vi "Login.vi"() -> ()   [LabVIEW 2015]
uses:
  <userlib>/QMH/Message Queue/Support/RunType.ctl
  <userlib>/QMH/Message Queue/Support/Enqueue Message (Single).vi
  <userlib>/QMH/Message Queue/Support/Enqueue Message (Array).vi
  <vilib>/Utility/error.llb/Error Cluster From Error Code.vi
  <userlib>/QMH/Message Queue/Support/Run Module(ref).vi
  <vilib>/ErrorRing/Error Ring.xnode
  <userlib>/QMH/User Event - Stop/User Event - Stop.lvlib
  <userlib>/QMH/Message Queue/Message Queue.lvlib
panel:
  in  "Authority":u16(ring) items=["学生", "老师"]
  in  "Login":bool
  in  "PassWord":string
  in  "用户名":string
  in  "Exit":bool
  in  "HostThread":variant
  # "权限 :"
  # "用户名 :"
  # "密码 :"
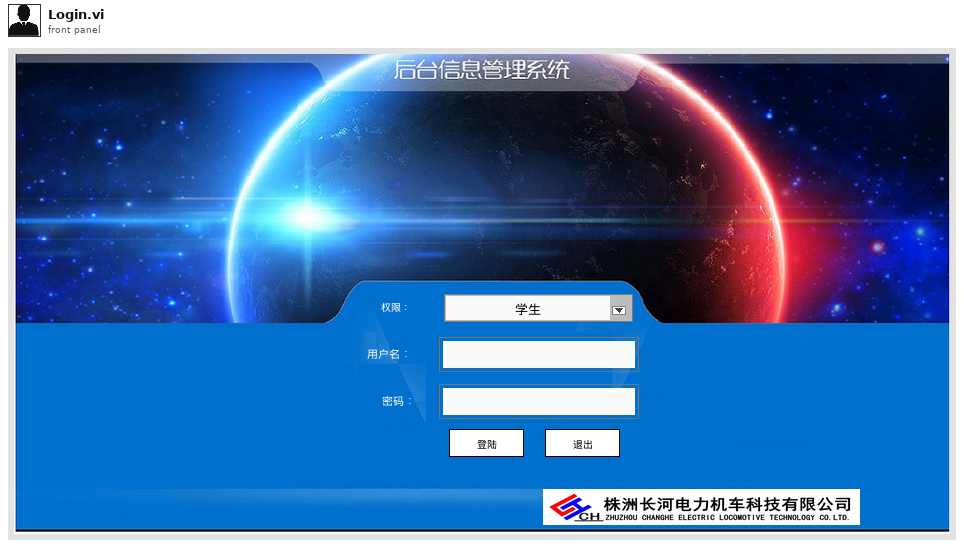
[diagram p1: front panel]
types:
  T1 = cluster{"Controls":cluster{"Exit":refnum<vi>, "Authority":refnum<vi>, "用户名":refnum<vi>, "密码":refnum<vi>}, "Thread":cluster{"ThisQ":string, "ThisVI":refnum<vi>, "HostQ":string, "HostRef":refnum<vi>, "SlavesQ":string[], "SlavesRef":refnum<vi>[]}, "Data":cluster{"Replace":bool}, "User":cluster{"Name":string}, "result?":bool, "Authority":u16}
  T2 = typedef "Message Queue.lvlib/RunType.ctl" = enum16{"Embeded", "Standard", "Hidden", "Minimized", "Maximzed", "RealTime"}
  T3 = cluster{"用户名":refnum<vi>, "密码":refnum<vi>, "Authority":refnum<vi>}
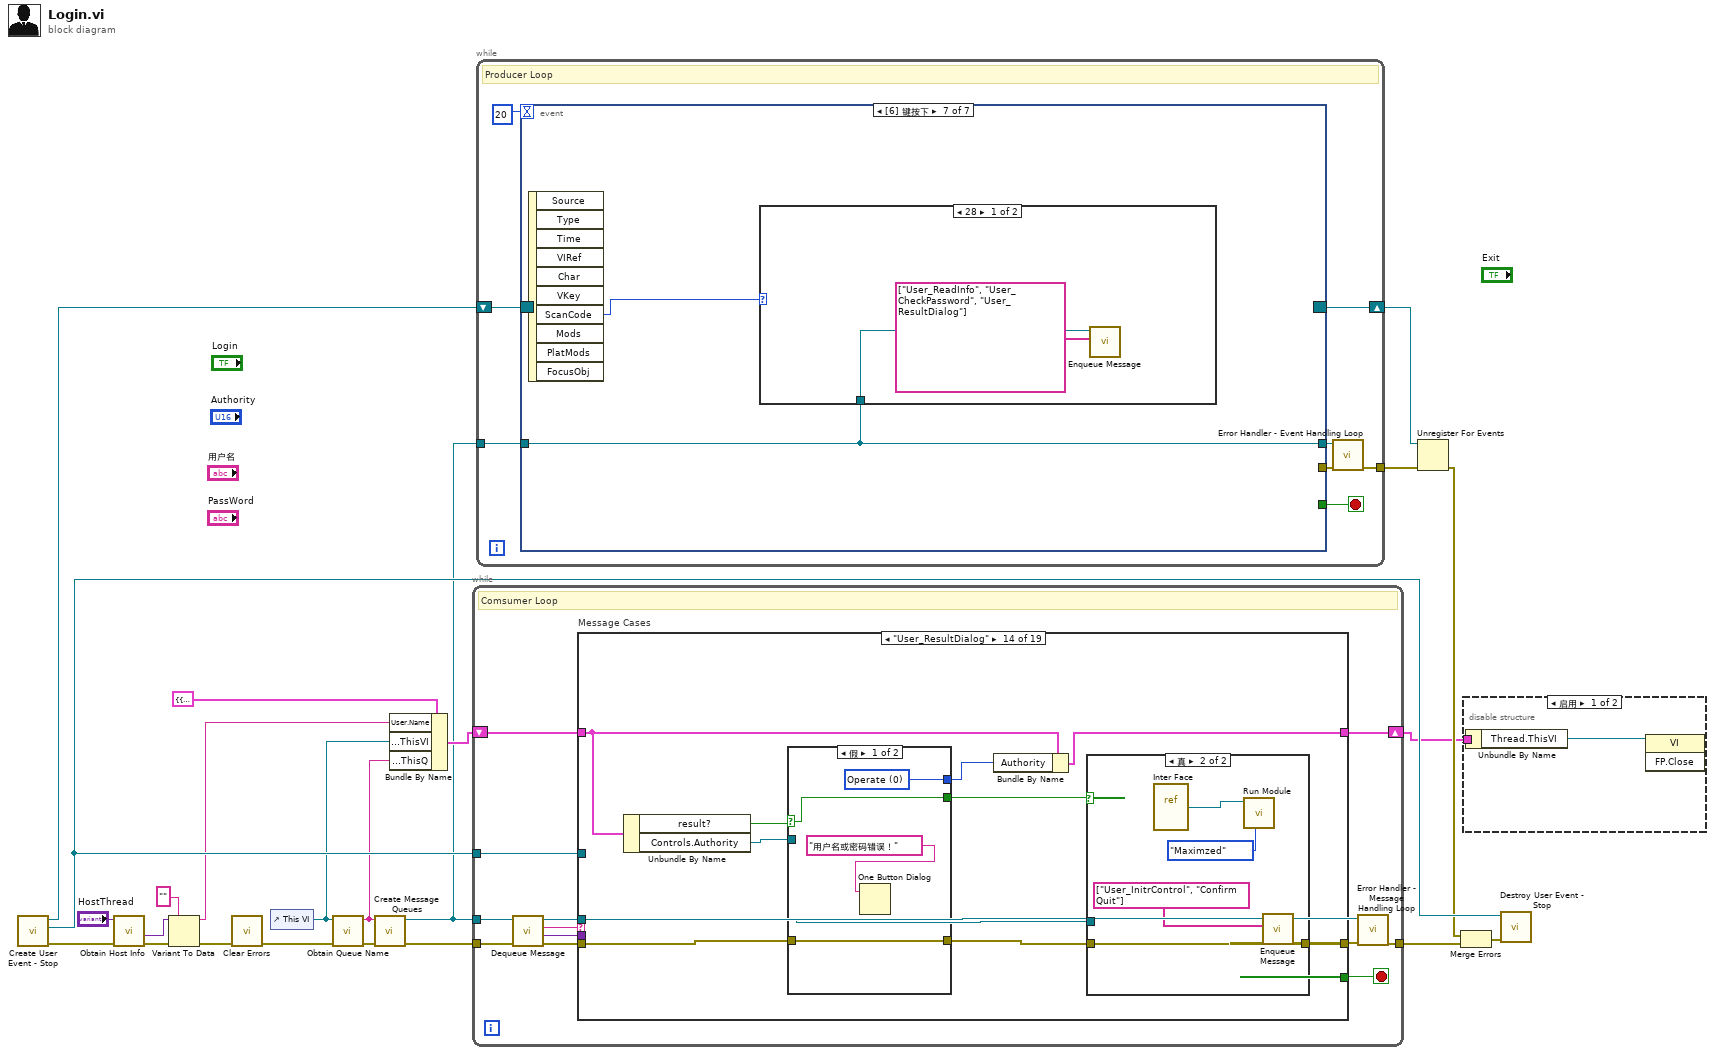
[diagram p0: block diagram]
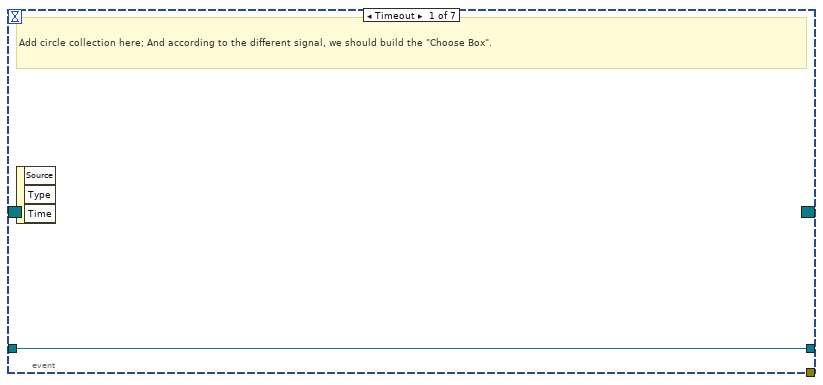
[diagram p3: hidden frame]
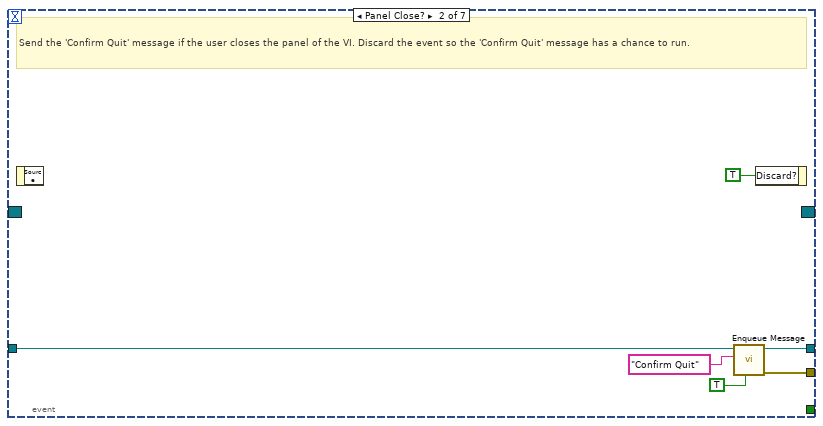
[diagram p4: hidden frame]
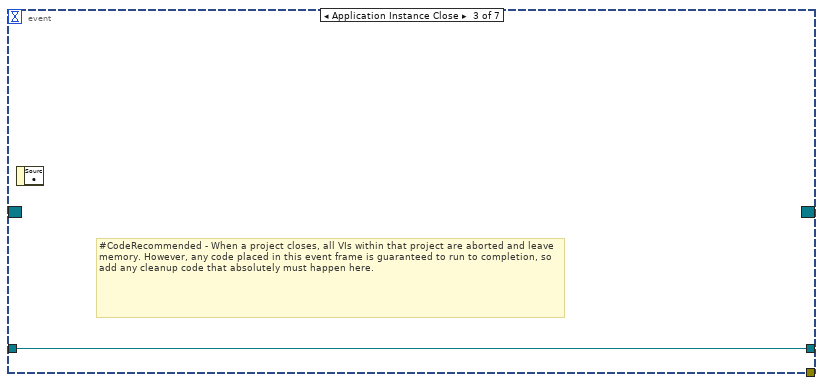
[diagram p5: hidden frame]
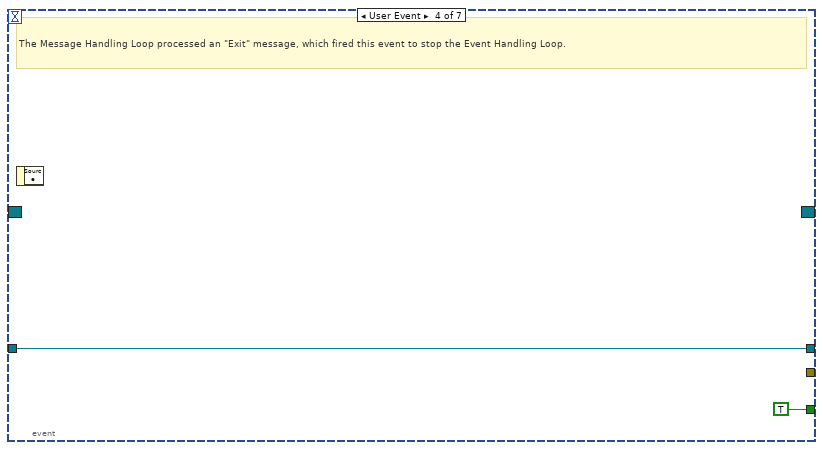
[diagram p6: hidden frame]
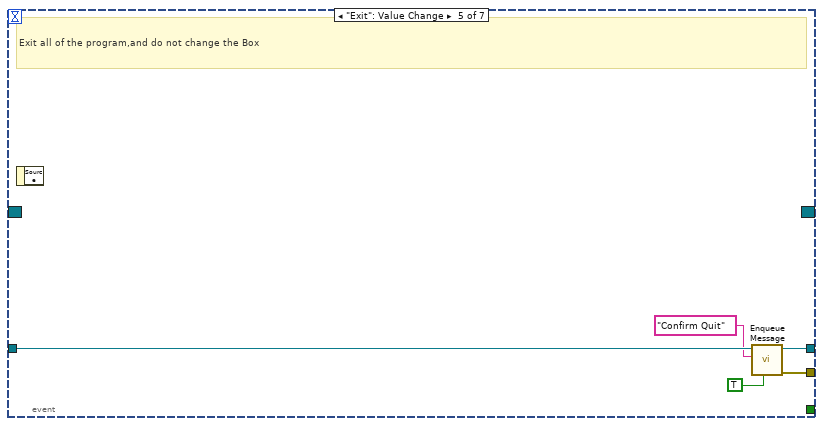
[diagram p7: hidden frame]
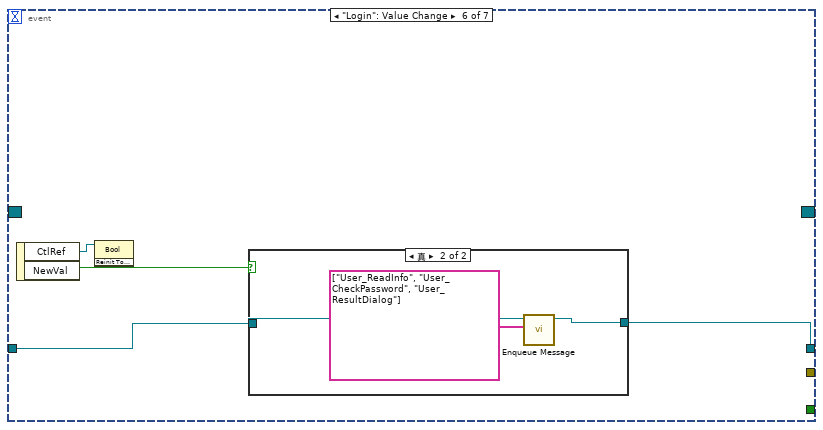
[diagram p8: hidden frame]
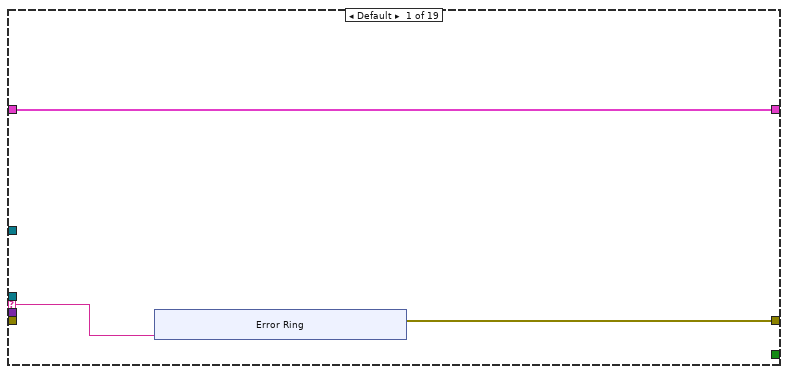
[diagram p11: hidden frame]
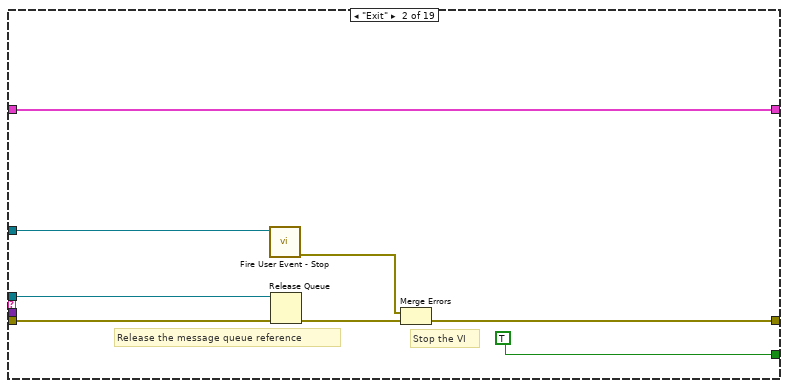
[diagram p12: hidden frame]
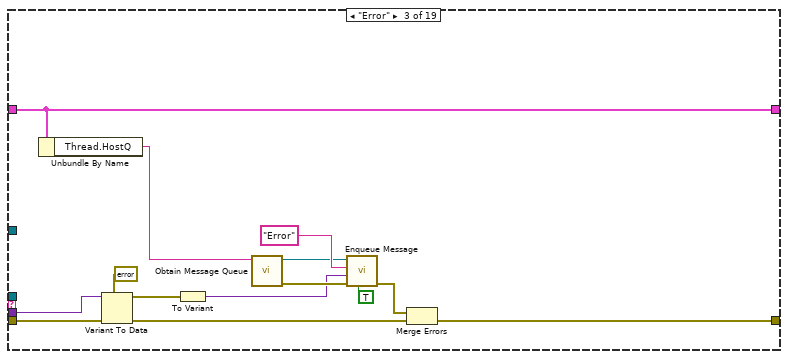
[diagram p13: hidden frame]
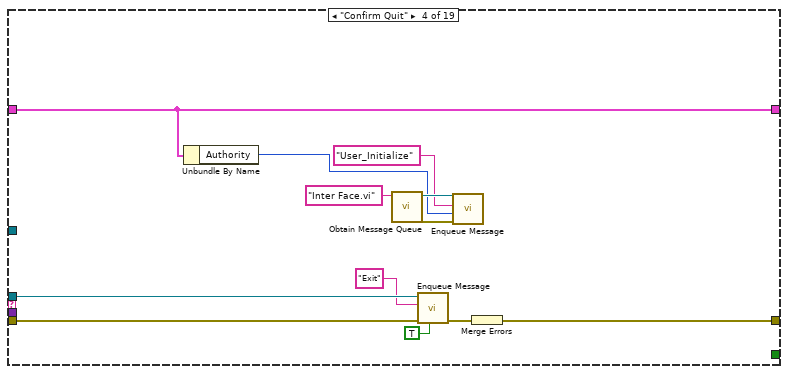
[diagram p14: hidden frame]
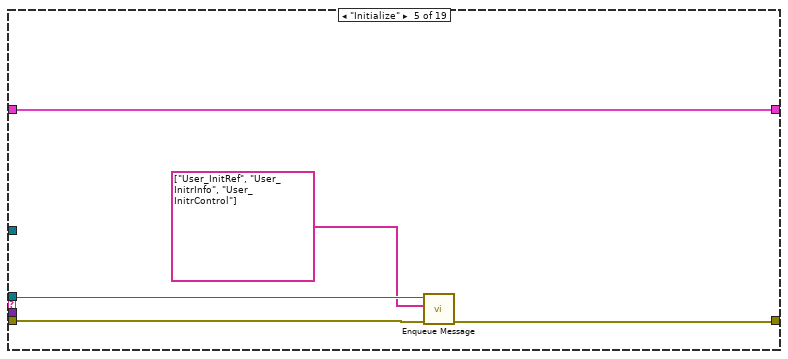
[diagram p15: hidden frame]
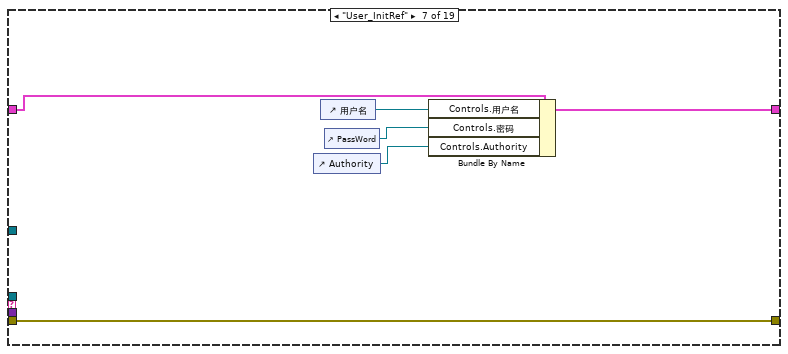
[diagram p17: hidden frame]
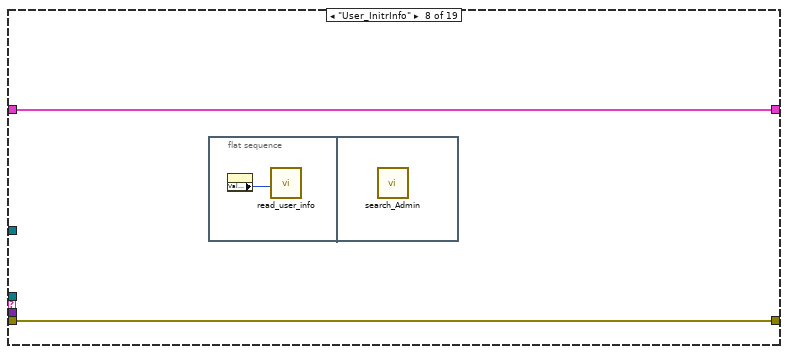
[diagram p18: hidden frame]
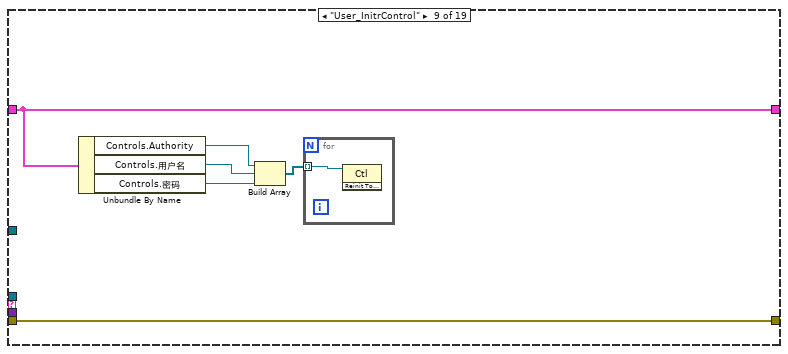
[diagram p19: hidden frame]
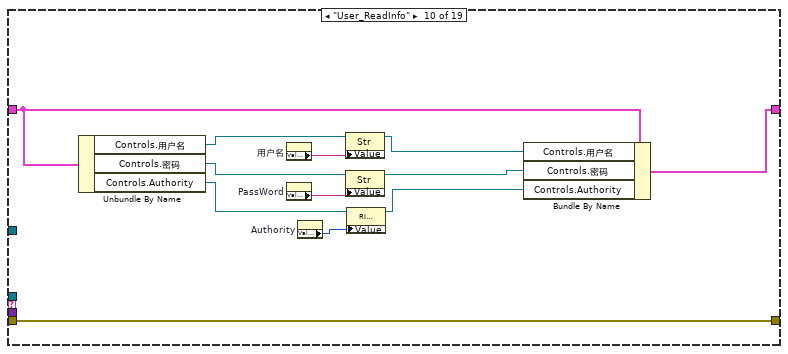
[diagram p20: hidden frame]
diagram:
  n1 = call <userlib>:"Create User Event - Stop.vi"() -> ("error out"=w10:errorcluster, "User Event - Stop"=w19:refnum<user-event>, "Stop Event Registration Refnum"=w21:refnum<event-registration>)  [unwired: 9 in]
  n2 = call <userlib>:"Obtain Host Info.vi"("error in (no error)"=w10, "HostThread"="HostThread") -> ("error out"=w7:errorcluster, "Data"=w6:variant)  [unwired: 6 in, 2 out]
  n3 = Variant To Data(error in=w7, type="", Variant=w6) -> (data=w2:string, error out=w4:errorcluster)
  n4 = call <vilib>:"Clear Errors.vi"("error in (no error)"=w4) -> ("error out"=w3:errorcluster)  [unwired: 5 in, 1 out]
  n5 = control-ref of="This VI"() -> (w12:refnum<vi>)
  n6 = call <userlib>:"Obtain Queue Name.vi"("error in (no error)"=w3, "VI Refnum"=w12) -> ("error out"=w15:errorcluster, "ViName"=w11:string)  [unwired: 8 in]
  n7 = call <userlib>:"Create Message Queues.vi"("error in (no error)"=w15, "name (unnamed)"=w11) -> ("error out"=w23:errorcluster, "QueueHandler"=w8:refnum<queue>)  [unwired: 8 in]
  n8 = Bundle By Name(cluster=T1 {"Controls"={"Exit"=refnum, "Authority"=refnum, "用户名"=refnum, "密码"=refnum}, "Thread"={"ThisQ"="", "ThisVI"=refnum, "HostQ"="", "HostRef"=refnum, "SlavesQ"=[], "SlavesRef"=[]}, "Data"={"Replace"=FALSE}, "User"={"Name"=""}, "result?"=FALSE, "Authority"=0} ("Data Cluster"), "User.Name"=w2, "Thread.ThisVI"=w12, "Thread.ThisQ"=w11) -> (w13:T1)
  n9 = while {
    tunnel: w8 -> [w27]
    shift-right: [w34] -> w1
    shift-left: w13 -> [w35]
    tunnel: w19 -> [w32]
    tunnel: w23 -> [w31]
    tunnel: [w25] -> w22
    stop <- w33 stop-if-true
    # "Comsumer Loop"
    n10 = call <userlib>:"Dequeue Message.vi"("error in (no error)"=w31, "Message Queue"=w27) -> ("error out"=w30:errorcluster, "Message Data"=w28:variant, "Message"=w29:string, "dup Message Queue"=w26:refnum<queue>)  [unwired: 6 in]
    n11 = case "Message Cases" shown="\"User_ResultDialog\"" w29 {
      selector: w29 -> [w36 _ _ _ _ _ _ _ _ _ _ _ _ _ _ _ _ _ _]
      tunnel: w26 -> [_ w53 _ w76 w81 _ _ _ _ _ _ _ _ w130 _ _ _ _ _]
      tunnel: w30 -> [_ w49 w67 w79 w83 w86 w92 w94 w101 w114 w122 w124 w126 w134 w153 w155 w157 w158 w161]
      tunnel: [w37 w50 w62 w78 w82 w86 w92 w94 w101 w114 w122 w124 w126 w132 w153 w155 w157 w158 w161] -> w24
      tunnel: w35 -> [w38 w46 w59 w69 w84 w85 w91 w93 w100 w113 w117 w123 w125 w129 w152 w154 w156 w159 w160]
      tunnel: [w38 w46 w59 w69 w84 w85 w90 w93 w100 w112 w116 w123 w125 w128 w152 w154 w156 w159 w160] -> w34
      tunnel: [_ TRUE _ _ _ _ _ _ _ _ _ _ _ _ _ _ _ _ _] -> w33
      tunnel: w28 -> [_ _ w66 _ _ _ _ _ _ _ _ _ _ _ _ _ _ _ _]
      tunnel: w32 -> [_ w48 _ _ _ _ _ _ _ _ _ _ _ _ _ _ _ _ _]
      frame Default {
        # "'Default' case only runs if there is a message that isn't defined in any of the other cases.  Output a programming error."
        n12 = xnode "Error Ring"("参数 0"=w36) -> ("错误输出"=w37:errorcluster)
      }
      frame "Exit" {
        # "Stop the VI"
        # "Release the message queue reference"
        # "Exit - Exit the application."
        n13 = call <userlib>:"Fire User Event - Stop.vi"("User Event - Stop"=w48) -> ("error out"=w47:errorcluster)  [unwired: 10 in]
        n14 = Release Queue(queue=w53, error in (no error)=w49) -> (error out=w51:errorcluster)  [unwired: 1 in, 2 out]
        n15 = Merge Errors(w47, w51) -> (w50:errorcluster)
      }
      frame "Error" {
        # "Error - Check the error message data and respond accordingly. This message is sent by the \"Error Handler\" VIs at the end of each loop in this application."
        n16 = Unbundle By Name(w59) -> ("Thread.HostQ"=w58:string)
        n17 = Variant To Data(error in=w67, type=errorcluster {"status"=FALSE, "code"=0, "source"=""} ("error constant"), Variant=w66) -> (data=w55:errorcluster, error out=w64:errorcluster)
        n18 = To Variant(anything=w55) -> (Variant=w54:variant)
        n19 = call <userlib>:"Obtain Message Queue.vi"("name (unnamed)"=w58) -> ("error out"=w57:errorcluster, "Message Queue"=w56:refnum<queue>)  [unwired: 9 in]
        n20 = call-poly <userlib>:"Enqueue Message.vi"("Priority Message? (F)"=TRUE, "error in (no error)"=w57, "Message Data"=w54, "Message"="Error", "Message Queue"=w56) -> ("error out"=w63:errorcluster)  [unwired: 5 in, 1 out]
        n21 = Merge Errors(w63, w64) -> (w62:errorcluster)
      }
      frame "Confirm Quit" {
        # "Confirm Quit - Message that can confirm whether or not the user wants to exit the application."
        n22 = Unbundle By Name(w69) -> ("Authority"=w68:u16)
        n23 = call <userlib>:"Obtain Message Queue.vi"("name (unnamed)"="Inter Face.vi") -> ("error out"=w70:errorcluster, "Message Queue"=w73:refnum<queue>)  [unwired: 9 in]
        n24 = call-poly <userlib>:"Enqueue Message.vi"("Priority Message? (F)"=TRUE, "error in (no error)"=w79, "Message"="Exit", "Message Queue"=w76) -> ("error out"=w77:errorcluster)  [unwired: 6 in, 1 out]
        n25 = call-poly <userlib>:"Enqueue Message.vi"("error in (no error)"=w70, "Message Data"=w68, "Message"="User_Initialize", "Message Queue"=w73) -> ()  [unwired: 6 in, 2 out]
        n26 = Merge Errors(w77) -> (w78:errorcluster)
      }
      frame "Initialize" {
        # "Initialize - Send separate messages to initialize the data and the front panel.  Bundle control references."
        n27 = call-poly <userlib>:"Enqueue Message.vi"("error in (no error)"=w83, "Message Array"=string[] ["User_InitRef", "User_InitrInfo", "User_InitrControl"], "Message Queue"=w81) -> ("error out"=w82:errorcluster)  [unwired: 7 in, 1 out]
      }
      frame "<------User------->" {
      }
      frame "User_InitRef" {
        n28 = control-ref of="Authority"() -> (w89:refnum<vi>)
        n29 = control-ref of="用户名"() -> (w88:refnum<vi>)
        n30 = control-ref of="PassWord"() -> (w87:refnum<vi>)
        n31 = Bundle By Name(cluster=w91, "Controls.用户名"=w88, "Controls.密码"=w87, "Controls.Authority"=w89) -> (w90:T1)
      }
      frame "User_InitrInfo" {
        n32 = flat-sequence {
          frame #0 {
            n33 = property on="Authority" class="Ring (严格)"() -> ("Value"=w95:u16)  [unwired: 2 in, 2 out]
            n34 = call "read_user_info.vi"("Authority"=w95) -> ()
          }
          frame #1 {
            n35 = call "search_Admin.vi"() -> ()  [unwired: 12 in]
          }
        }
      }
      frame "User_InitrControl" {
        n36 = Unbundle By Name(w100) -> ("Controls.Authority"=w99:refnum<vi>, "Controls.用户名"=w98:refnum<vi>, "Controls.密码"=w97:refnum<vi>)
        n37 = Build Array(w99, w98, w97) -> (w96:refnum<vi>[])
        n38 = for {
          tunnel: w96 -> [w102] mode=indexing
          n39 = invoke class="Ctl" method="Reinit To Default"(reference=w102) -> ()  [unwired: 2 in, 3 out]
        }
      }
      frame "User_ReadInfo" {
        n40 = Unbundle By Name(w113) -> ("Controls.用户名"=w108:refnum<vi>, "Controls.密码"=w107:refnum<vi>, "Controls.Authority"=w106:refnum<vi>)
        n41 = property on="用户名" class="Str"() -> ("Value"=w104:string)  [unwired: 2 in, 2 out]
        n42 = property on="PassWord" class="Str"() -> ("Value"=w103:string)  [unwired: 2 in, 2 out]
        n43 = property on="Authority" class="Ring (严格)"() -> ("Value"=w105:u16)  [unwired: 2 in, 2 out]
        n44 = property class="Str"(reference=w108, "Value"=w104) -> (reference out=w111:refnum<vi>)  [unwired: 1 in, 1 out]
        n45 = property class="Str"(reference=w107, "Value"=w103) -> (reference out=w110:refnum<vi>)  [unwired: 1 in, 1 out]
        n46 = property class="Ring (严格)"(reference=w106, "Value"=w105) -> (reference out=w109:refnum<vi>)  [unwired: 1 in, 1 out]
        n47 = Bundle By Name(cluster=w113, "Controls.用户名"=w111, "Controls.密码"=w110, "Controls.Authority"=w109) -> (w112:T1)
      }
      frame "User_CheckPassword" {
        n48 = Unbundle By Name(w117) -> ("Controls.用户名"=w121:refnum<vi>, "Controls.密码"=w120:refnum<vi>, "Controls.Authority"=w119:refnum<vi>)
        n49 = Bundle("用户名"=w121, "密码"=w120, "Authority"=w119) -> (w118:T3)  [unwired: 1 in]
        n50 = call "check_password.vi"("Ref"=w118) -> ("result？"=w115:bool)
        n51 = Bundle By Name(cluster=w117, "result?"=w115) -> (w116:T1)
      }
      frame "User_Add" {
      }
      frame "User_Delete" {
      }
      frame "User_ResultDialog" {
        n52 = Unbundle By Name(w129) -> ("result?"=w136:bool, "Controls.Authority"=w135:refnum<vi>)
        n53 = case shown="假" w136 {
          selector: w136 -> [w146 w150]
          tunnel: w135 -> [_ w151]
          tunnel: w134 -> [w147 w149]
          tunnel: [w147 w149] -> w131
          tunnel: [w146 w150] -> w133
          tunnel: [w145 w148] -> w127
          frame False {
            w145 = u16 0 items=["Operate", "Tech", "Supervisor", "Admin"] ("Authority_In")
            n54 = One Button Dialog(message="用户名或密码错误！" ("Message")) -> ()  [unwired: 1 in, 1 out]
          }
          frame True {
            n55 = property class="Ring (严格)"(reference=w151) -> ("Value"=w148:u16)  [unwired: 1 in, 2 out]
          }
        }
        n56 = Bundle By Name(cluster=w129, "Authority"=w127) -> (w128:T1)
        n57 = case shown="真" w133 {
          tunnel: [w137 w138] -> w132
          tunnel: w131 -> [w137 w139]
          tunnel: w130 -> [_ w140]
          frame False {
          }
          frame True {
            n58 = vi-ref "Inter Face.vi"() -> (w143:refnum<vi>)
            n59 = call-poly <userlib>:"Run Module.vi"("Type"=RunType."Maximzed", "VI Ref in"=w143) -> ()  [unwired: 7 in, 3 out]
            n60 = call-poly <userlib>:"Enqueue Message.vi"("error in (no error)"=w139, "Message Array"=string[] ["User_InitrControl", "Confirm Quit"], "Message Queue"=w140) -> ("error out"=w138:errorcluster)  [unwired: 7 in, 1 out]
          }
        }
      }
      frame "<-------UI-------->" {
      }
      frame "Init_controls" {
      }
      frame "<------Core------>" {
      }
      frame "Core_InitializeRef" {
        # "Initialize control references. For there is not enough space to locate all the control references, separate the codes into 2 messages"
      }
      frame "<---Operation--->" {
      }
    }
    n61 = call <userlib>:"Error Handler - Message Handling Loop.vi"("error in (no error)"=w24, "Message Queue"=w26) -> ("dup error in"=w25:errorcluster)  [unwired: 8 in, 1 out]
  }
  n62 = while {
    tunnel: w8 -> [w169]
    shift-right: [w167] -> w17
    shift-left: w21 -> [w168]
    tunnel: [w163] -> w16
    stop <- w165 stop-if-true
    # "Producer Loop"
    n63 = event shown="[6] 键按下" {
      selector: w168 -> [_ _ _ _ _ _ _]
      dyn-events: [_ _ _ _ _ _ _] -> w167
      timeout: 20 -> [_ _ _ _ _ _ _]
      tunnel: [_ _ _ TRUE ("Discard?") _ _ _] -> w165
      tunnel: w169 -> [w170 w175 w177 w179 w184 w188 w193]
      tunnel: [_ w174 _ _ w182 _ _] -> w166
      tunnel: [w170 w173 w177 w179 w183 w187 w193] -> w164
      event Timeout {
        # "Add circle collection here; And according to the different signal, we should build the \"Choose Box\"."
        n64 = event-data() -> ()  [unwired: 1 in, 3 out]
      }
      event Panel Close? {
        # "Send the 'Confirm Quit' message if the user closes the panel of the VI. Discard the event so the 'Confirm Quit' message has a chance to run."
        n65 = event-data() -> ()  [unwired: 1 in, 1 out]
        n66 = call-poly <userlib>:"Enqueue Message.vi"("Priority Message? (F)"=TRUE, "Message"="Confirm Quit", "Message Queue"=w175) -> ("error out"=w174:errorcluster, "dup Message Queue"=w173:refnum<queue>)  [unwired: 7 in]
        n67 = event-data("Discard?"=TRUE) -> ()  [unwired: 1 in, 1 out]
      }
      event Application Instance Close {
        # "#CodeRecommended - When a project closes, all VIs within that project are aborted and leave memory. However, any code placed in this event frame is guaranteed to run to completion, so add any cleanup code that absolutely must happen here."
        n68 = event-data() -> ()  [unwired: 1 in, 1 out]
      }
      event User Event {
        # "The Message Handling Loop processed an \"Exit\" message, which fired this event to stop the Event Handling Loop."
        n69 = event-data() -> ()  [unwired: 1 in, 1 out]
      }
      event "Exit": Value Change {
        # "Exit all of the program,and do not change the Box"
        n70 = event-data() -> ()  [unwired: 1 in, 1 out]
        n71 = call-poly <userlib>:"Enqueue Message.vi"("Priority Message? (F)"=TRUE, "Message"="Confirm Quit", "Message Queue"=w184) -> ("error out"=w182:errorcluster, "dup Message Queue"=w183:refnum<queue>)  [unwired: 7 in]
      }
      event "Login": Value Change {
        n72 = event-data() -> ("CtlRef"=w185:refnum<vi>, "NewVal"=w186:bool)  [unwired: 1 in]
        n73 = invoke class="Bool" method="Reinit To Default"(reference=w185) -> ()  [unwired: 2 in, 3 out]
        n74 = case shown="真" w186 {
          tunnel: w188 -> [w189 w192]
          tunnel: [w189 w191] -> w187
          frame False {
          }
          frame True {
            n75 = call-poly <userlib>:"Enqueue Message.vi"("Message Array"=string[] ["User_ReadInfo", "User_CheckPassword", "User_ResultDialog"], "Message Queue"=w192) -> ("dup Message Queue"=w191:refnum<queue>)  [unwired: 8 in, 1 out]
          }
        }
      }
      event Key Down {
        n76 = event-data() -> ("ScanCode"=w194:i16)  [unwired: 1 in, 9 out]
        n77 = case shown="28" w194 {
          tunnel: w193 -> [w195 _]
          frame 28 {
            n78 = call-poly <userlib>:"Enqueue Message.vi"("Message Array"=string[] ["User_ReadInfo", "User_CheckPassword", "User_ResultDialog"], "Message Queue"=w195) -> ()  [unwired: 8 in, 2 out]
          }
          frame 0, Default {
          }
        }
      }
    }
    n79 = call <userlib>:"Error Handler - Event Handling Loop.vi"("error in (no error)"=w166, "Message Queue"=w164) -> ("dup error in"=w163:errorcluster)  [unwired: 8 in, 1 out]
  }
  n80 = Unregister For Events(event registration refnum=w17, error in=w16) -> (error out=w18:errorcluster)
  n81 = Merge Errors(w18, w22) -> (w20:errorcluster)
  n82 = disable-structure shown="启用" {
    disable-tunnel: w1 -> [w198 _]
    frame Enabled {
      n83 = Unbundle By Name(w198) -> ("Thread.ThisVI"=w197:refnum<vi>)
      n84 = invoke class="VI" method="FP.Close"(reference=w197) -> ()  [unwired: 2 in, 3 out]
    }
    frame Disabled {
    }
  }
  n85 = call <userlib>:"Destroy User Event - Stop.vi"("error in (no error)"=w20, "User Event - Stop"=w19) -> ()  [unwired: 9 in, 1 out]
